vi "Custom Symbols--constant.vi"() -> (3 "Custom Symbols":cluster{"Symbol Paths":path[], "IDs":string[]}={"Symbol Paths"=[path "../resource/Framework/Providers/Icons/VI.png", path "../resource/Framework/Providers/Icons/vim.png", path "../resource/Framework/Providers/Icons/vit.png", path "../resource/Framework/Providers/Icons/UDClass VI.png", path "../resource/Framework/Providers/Icons/UDClass.png", path "../resource/Framework/Providers/Icons/lvlib.png", path "../resource/Framework/Providers/Icons/MyComputer.png", path "../resource/Framework/Providers/Icons/lvrt_pxi.png", path "../resource/Framework/Providers/Icons/Folder.png"], "IDs"=["vi", "vim", "vit", "class_vi", "lvclass", "lvlib", "My Computer", "Target", "Folder"]})   [LabVIEW 2020, in "Project Tree.lvlib" / "Project Tree Map.lvclass"]
uses:
  Project Tree Map.lvclass
  Project Tree Map.lvclass/Project Tree Map.ctl
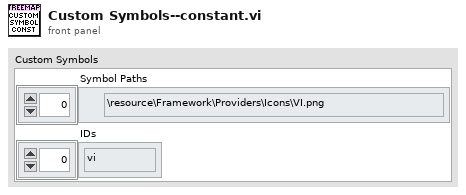
[diagram p1: front panel]
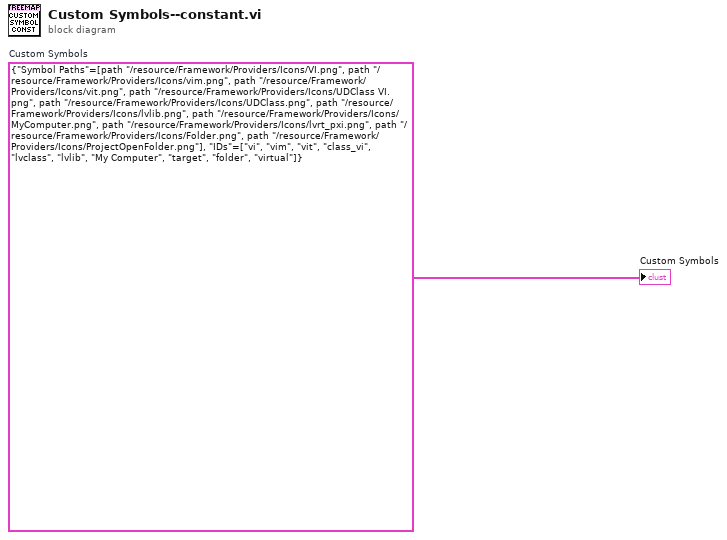
[diagram p0: block diagram]
diagram:
  w1 = cluster{"Symbol Paths":path[], "IDs":string[]} {"Symbol Paths"=[path "../resource/Framework/Providers/Icons/VI.png", path "../resource/Framework/Providers/Icons/vim.png", path "../resource/Framework/Providers/Icons/vit.png", path "../resource/Framework/Providers/Icons/UDClass VI.png", path "../resource/Framework/Providers/Icons/UDClass.png", path "../resource/Framework/Providers/Icons/lvlib.png", path "../resource/Framework/Providers/Icons/MyComputer.png", path "../resource/Framework/Providers/Icons/lvrt_pxi.png", path "../resource/Framework/Providers/Icons/Folder.png", path "../resource/Framework/Providers/Icons/ProjectOpenFolder.png"], "IDs"=["vi", "vim", "vit", "class_vi", "lvclass", "lvlib", "My Computer", "target", "folder", "virtual"]}  # Custom Symbols
  "Custom Symbols" <- w1
